vi "Resync_OpalRT_LC.vi"() -> ()   [LabVIEW 2016]
uses:
  LabVIEW Data/MathScriptVIs/MCStatic_36913154532_6c89d161b761586b3ea5426e3c3dd88c.vi
  <instcachedir>/0/MCStatic_36913154532_6c89d161b761586b3ea5426e3c3dd88c_A126C061F6454585938C826FD07650FA.lvgen/MCStatic_36913154532_6c89d161b761586b3ea5426e3c3dd88c_A126C061F6454585938C826FD07650FA_002.vi
  <vilib>/imath/engines/lvmath2/RunTimeEngine/NodeEndStatement/NIMS_NodeEndStatement_Output.vi
  <instcachedir>/0/NIMS_NodeEndStatement_Output_53EC0D466D134D7ABD903AC30B43404B.lvgen/NIMS_NodeEndStatement_Output_53EC0D466D134D7ABD903AC30B43404B_001.vi
  <vilib>/imath/engines/lvmath2/RunTimeEngine/ErrorHandling/NIMS_Finalize Error.vi
  LCs_forRTDS/Dependencies/PIcontroller.m
panel:
  out "error out":errorcluster
  in  "i_an":dbl=0.09999999999999964
  in  "p_an":dbl=0.20000000000000018
  in  "i_in":dbl=4.1
  in  "p_in":dbl=3.0999999999999996
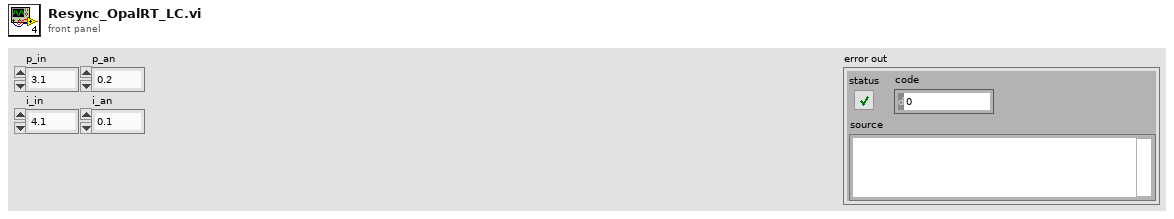
[diagram p1: front panel]
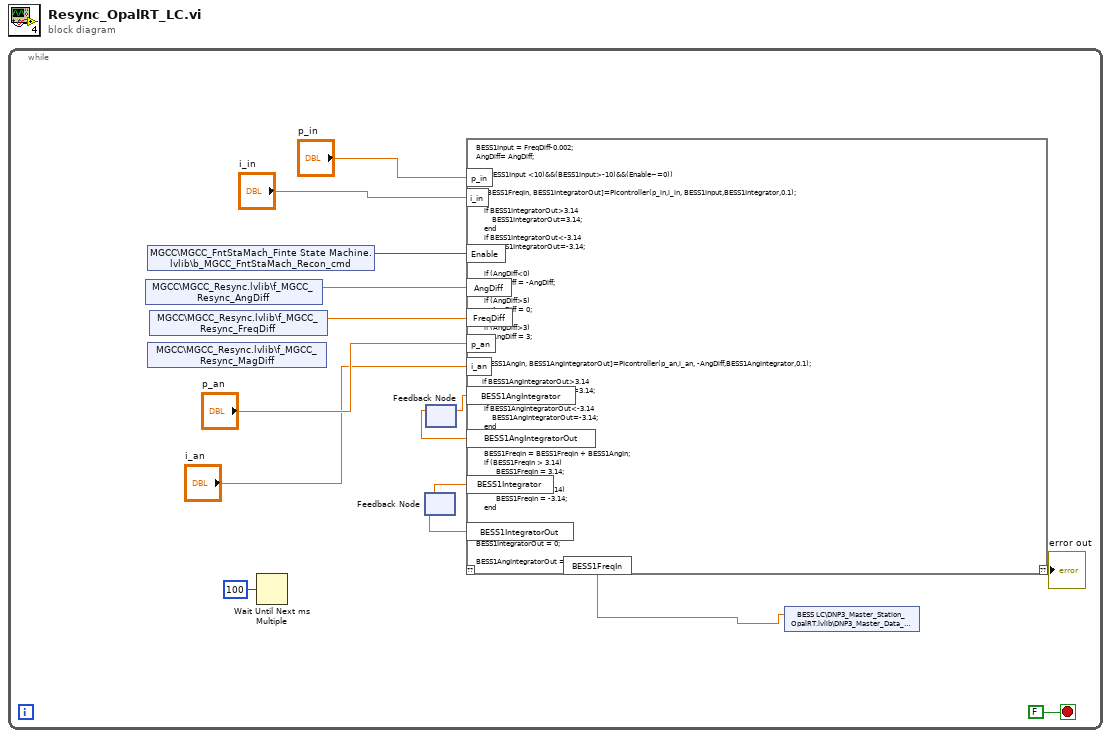
[diagram p0: block diagram]
diagram:
  n1 = while {
    stop <- FALSE stop-if-true
    n2 = shared-variable "MGCC\\MGCC_Resync.lvlib\\f_MGCC_Resync_AngDiff"() -> (w13:dbl)  [unwired: 1 in, 1 out]
    n3 = shared-variable "MGCC\\MGCC_FntStaMach_Finte State Machine.lvlib\\b_MGCC_FntStaMach_Recon_cmd"() -> (w9:bool)  [unwired: 1 in, 1 out]
    n4 = shared-variable "MGCC\\MGCC_Resync.lvlib\\f_MGCC_Resync_MagDiff"() -> ()  [unwired: 1 in, 2 out]
    n5 = shared-variable "MGCC\\MGCC_Resync.lvlib\\f_MGCC_Resync_FreqDiff"() -> (w12:dbl)  [unwired: 1 in, 1 out]
    n6 = Wait Until Next ms Multiple(millisecond multiple=u32 100) -> ()  [unwired: 1 out]
    n7 = feedback #1() -> (w15:dbl)  [unwired: 1 in]
    n8 = feedback #2() -> (w10:dbl)  [unwired: 1 in]
    n9 = mathscript code="BESS1Input = FreqDiff-0.002;\nAngDiff= AngDiff;\n\nif ((BESS1Input <10)&&(BESS1Input>-10)&&(Enable~=0))\n\n    [BESS1FreqIn, BESS1IntegratorOut]=PIcontroller(p_in,i_in, BESS1Input,BESS1Integrator,0.1);\n   \n    if BESS1IntegratorOut>3.14\n        BESS1IntegratorOut=3.14;\n    end\n    if BESS1IntegratorOut<-3.14\n        BESS1IntegratorOut=-3.14;\n    end\n\n    if (AngDiff<0)\n        AngDiff = -AngDiff;\n    end \n    if (AngDiff>5)\n        AngDiff = 0;\n    end \n    if (AngDiff>3)\n        AngDiff = 3;\n    end \n\n   [BESS1AngIn, BESS1AngIntegratorOut]=PIcontroller(p_an,i_an, -AngDiff,BESS1AngIntegrator,0.1);\n\n   if BESS1AngIntegratorOut>3.14\n        BESS1AngIntegratorOut=3.14;\n    end\n    if BESS1AngIntegratorOut<-3.14\n        BESS1AngIntegratorOut=-3.14;\n    end\n    \n\n    BESS1FreqIn = BESS1FreqIn + BESS1AngIn;\n    if (BESS1FreqIn > 3.14) \n          BESS1FreqIn = 3.14;\n    end\n    if (BESS1FreqIn < -3.14) \n          BESS1FreqIn = -3.14;\n    end\n\nelse\nBESS1FreqIn = 0;\nBESS1IntegratorOut = 0;\n\nBESS1AngIntegratorOut = 0;\nend"("AngDiff"=w13, "BESS1Integrator"=w15, "FreqDiff"=w12, "BESS1AngIntegrator"=w10, "Enable"=w9, "p_in"="p_in", "i_in"="i_in", "p_an"="p_an", "i_an"="i_an") -> ("??"=→"error out":errorcluster, "BESS1IntegratorOut"=w14:dbl, "BESS1FreqIn"=w6:dbl, "BESS1AngIntegratorOut"=w11:dbl)  [unwired: 1 in]
    n10 = feedback-in #1(w14) -> ()
    n11 = feedback-in #2(w11) -> ()
    n12 = shared-variable "BESS LC\\DNP3_Master_Station_OpalRT.lvlib\\DNP3_Master_Data_Variables.lvlib\\MS_Analog_Control.lvlib\\BESS-FREQ-CMD"(w6) -> ()  [unwired: 1 in, 1 out]
  }
